vi "MMC_COM_open.vi"(3 "COM port select":u8=1) -> (0 "Error out":errorcluster, 1 "function return":i32)   [LabVIEW 2024]
doc: "This vi oprns the RS-232 port for Mercury communications"
uses:
  MMC.dll
panel:
  out "Message":string
  # "MMC_COM_open"
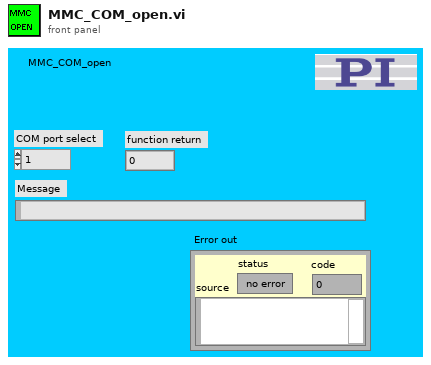
[diagram p1: front panel]
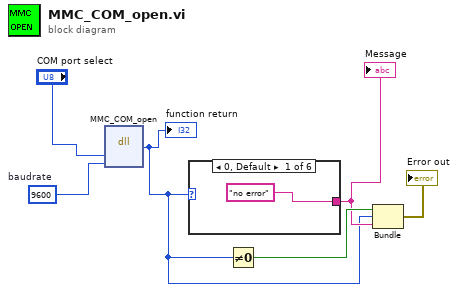
[diagram p0: block diagram]
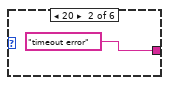
[diagram p2: hidden frame]
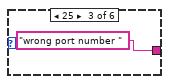
[diagram p3: hidden frame]
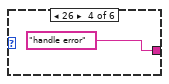
[diagram p4: hidden frame]
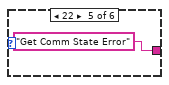
[diagram p5: hidden frame]
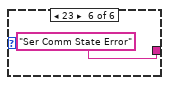
[diagram p6: hidden frame]
diagram:
  w6 = 9600  # baudrate
  n1 = dll-call lib="E:/Wilson/HoppingSICM_TK/HoppingSICM_v2/DLLs/MMC.dll" fn="MMC_COM_open"("portnumber"="COM port select", "baudrate"=w6) -> ("return type"=w2:i32)  [unwired: 5 in, 2 out]
  "function return" <- w2
  n2 = case shown="0, Default" w2 {
    tunnel: ["no error" "timeout error" "wrong port number " "handle error" "Get Comm State Error" "Ser Comm State Error"] -> w3
    frame 0, Default {
    }
    frame 20 {
    }
    frame 25 {
    }
    frame 26 {
    }
    frame 22 {
    }
    frame 23 {
    }
  }
  "Message" <- w3
  n3 = Not Equal To 0?(x=w2) -> (x != 0?=w4:bool)
  n4 = Bundle(w4, "return type"=w2, w3) -> (→"Error out":cluster{bool, "return type":i32, string})  [unwired: 1 in]
